vi "GetElapsedTandFPS-1.vi"(5 "[IN] Timer Count Before ALL [ms]":u32, 6 "[IN] Timer Count After ALL [ms]":u32) -> (0 "[OUT] Raw FPS":dbl, 1 "[OUT] Rounded FPS":u16, 2 "[OUT] Elapsed time [ms]":u32)   [LabVIEW 2020]
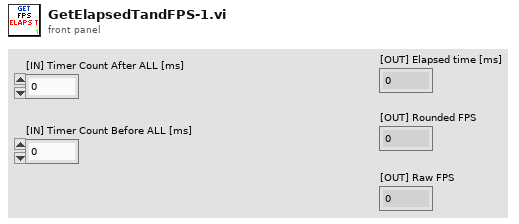
[diagram p1: front panel]
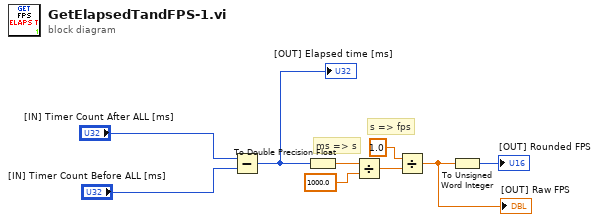
[diagram p0: block diagram]
diagram:
  # "s => fps"
  # "ms => s"
  n1 = Subtract(x="[IN] Timer Count After ALL [ms]", y="[IN] Timer Count Before ALL [ms]") -> (x-y=w2:u32)
  "[OUT] Elapsed time [ms]" <- w2
  n2 = To Double Precision Float(number=w2) -> (double precision float=w7:dbl)
  n3 = Divide(x=w7, y=1000.0) -> (x/y=w5:dbl)
  n4 = Divide(x=1.0, y=w5) -> (x/y=w3:dbl)
  "[OUT] Raw FPS" <- w3
  n5 = To Unsigned Word Integer(number=w3) -> (unsigned 16bit integer=→"[OUT] Rounded FPS":u16)
